vi "Drive_PositionControl.vi"(8 "error in":errorcluster, 9 "Speed limit":dbl, 10 "Right_Distance":dbl, 11 "Left_Distance":dbl) -> (0 "error out":errorcluster)   [LabVIEW 2009, in "Drive.lvlib"]
doc: "This VI implements position control of the robot drive using set speed function. It contains loop inside that runs until desired position is reached. So do not use this VI in the outer while loop directly. This VI also ramps up speed of the robot to make position control more accurate.\n\nThe VI requires desired distances to travel for both left and right sides of the robot as inputs.\nSpeed input value limits the speed of the robot during movement.\n\nTo abort the execution, use \"Drive_StopDrive\" VI and set input \"Abort?\" to true.\nTo straight forward movement, input the same value to both distances.\nTo turn on spot, input opposite values to distances.\nDifferent values will cause the robot to move along arc with some radius."
uses:
  Drive.lvlib
  <vilib>/Platform/TimedLoop/XDataNode/XDataNode.xnode
  <vilib>/Platform/TimedLoop/XDataNode/loadlvalarms.vi
  <vilib>/Platform/TimedLoop/XDataNode/timing_clust.ctl
  <vilib>/Platform/TimedLoop/XDataNode/nitl_modes.ctl
  <vilib>/Platform/TimedLoop/XDataNode/wakeup.ctl
  Drive_Utils_CalculateSpeed.vi
  Drive_ControlMode.ctl
  <vilib>/Platform/TimedLoop/XDataNode/XDNodeRunTimeDep.lvlib
  Drive_Utils.lvlib
  Utility.lvlib
panel:
  out "state out":T1
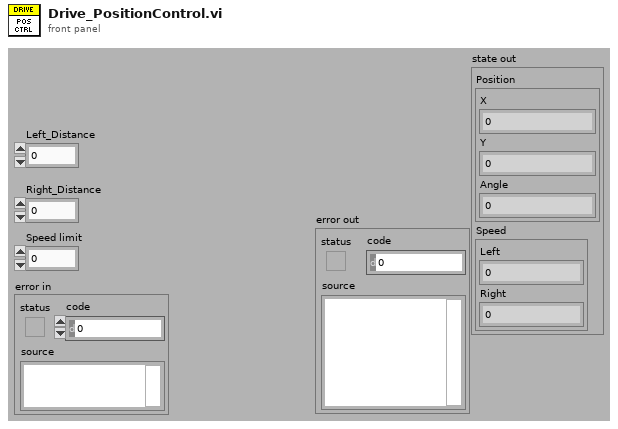
[diagram p1: front panel]
types:
  T1 = cluster{"Position":cluster{"X":dbl, "Y":dbl, "Angle":dbl}, "Speed":cluster{"Left":dbl, "Right":dbl}}
  T2 = typedef "XDNodeRunTimeDep.lvlib/timing_clust.ctl" = cluster{"Expected End [f-1]":u64, "Actual End [f-1]":u64, "Finished Late? [f-1]":bool, "Expected End [i-1]":u64, "Actual End [i-1]":u64, "Finished Late? [i-1]":bool, "Expected Start [i]":u64, "Actual Start [i]":u64, "Expected Start [f]":u64, "Actual Start [f]":u64, "Source Name":string, "Structure Name":string, "Period":i64, "Deadline":i64, "Offset":i64, "Start":i64, "Priority":i32, "Timeout":i32, "Mode":T3, "Wakeup Reason":T4, "Error":errorcluster, "Source Type":string, "Secondary Source Type":string, "Global End Time":u64, "Global Start Time":u64, "Frame Duration":u64, "Iteration Duration":u64, "Assigned CPU":i32, "I/O Scan Engine Mode":u32}
  T3 = typedef "XDNodeRunTimeDep.lvlib/nitl_modes.ctl" = enum32{"No Change", "Process missed periods, maintain original phase", "Discard missed periods, maintain original phase", "Process missed periods, ignore original phase", "Discard missed periods, ignore original phase"}
  T4 = typedef "XDNodeRunTimeDep.lvlib/wakeup.ctl" = enum32{"Normal", "Aborted", "Asynchronous wakeup", "Timing source error", "Timed loop error", "Timeout"}
  T5 = typedef "Drive.lvlib/Drive_ControlMode.ctl" = enum16{"CAN", "PWM"}
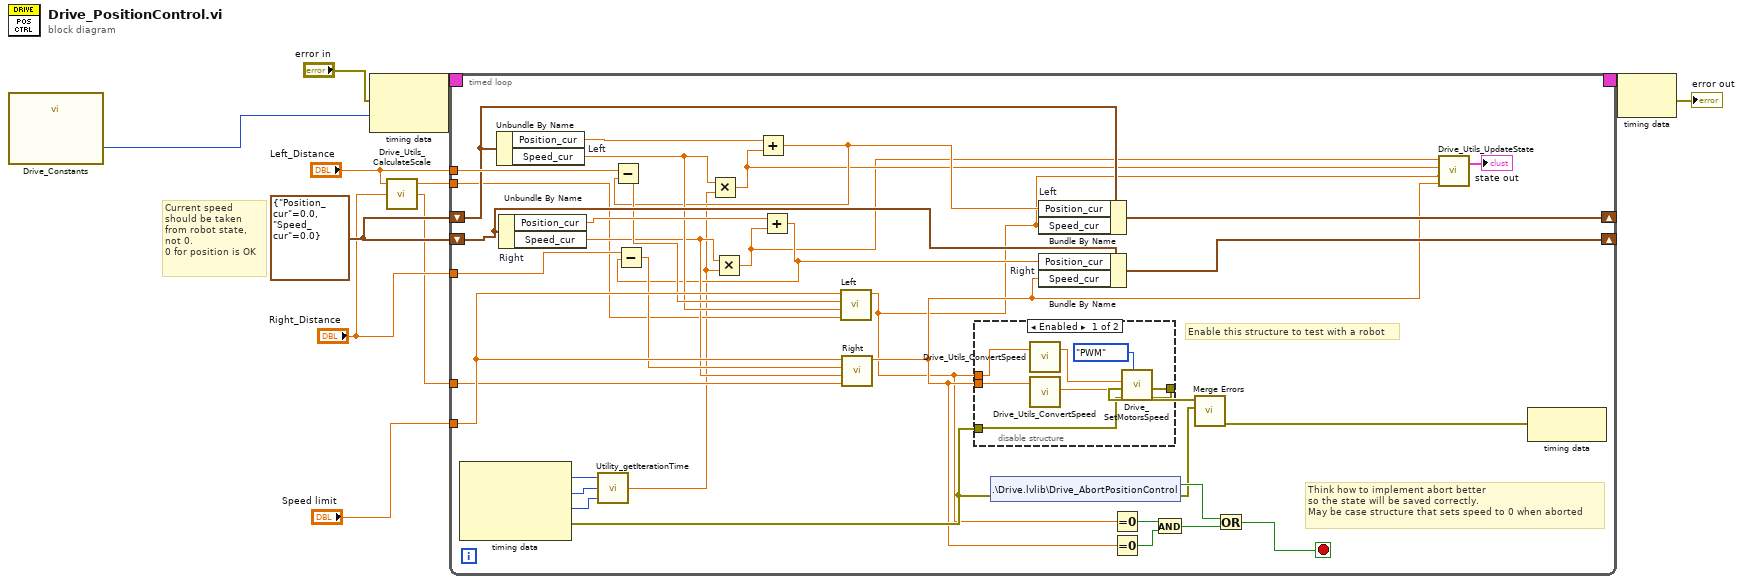
[diagram p0: block diagram]
diagram:
  w6 = cluster{"Position_cur":dbl, "Speed_cur":dbl} {"Position_cur"=0.0, "Speed_cur"=0.0}
  # "Current speed\nshould be taken\nfrom robot state,\nnot 0.\n0 for position is OK"
  n1 = call "Drive_Constants.vi"() -> ("Position control loop period (ms)"=w1:i64)  [unwired: 23 in, 4 out]
  n2 = node-c288("error in", w1) -> (w11:T2)
  n3 = call "Drive_Utils_CalculateScale.vi"("Right distance"="Right_Distance", "Left distance"="Left_Distance") -> ("Right scale"=w2:dbl, "Left scale"=w3:dbl)  [unwired: 1 in, 1 out]
  n4 = timed-loop {
    timing: w11 -> [_]
    timing-out: [_] -> w10
    tunnel: "Left_Distance" -> [w46]
    shift-right: [w43] -> _
    shift-left: w6 -> [w44]
    shift-right: [w40] -> _
    shift-left: w6 -> [w39]
    tunnel: "Right_Distance" -> [w42]
    tunnel: "Speed limit" -> [w38]
    tunnel: w3 -> [w29]
    tunnel: w2 -> [w28]
    stop <- w25 stop-if-true
    # "Enable this structure to test with a robot"
    # "Think how to implement abort better\nso the state will be saved correctly.\nMay be case structure that sets speed to 0 when aborted"
    n5 = node-c288() -> (w23:i64, w22:i64, w21:i64, w20:errorcluster)  [unwired: 1 in]
    n6 = Unbundle By Name "Left"(w44) -> ("Position_cur"=w45:dbl, "Speed_cur"=w35:dbl)
    n7 = Unbundle By Name "Right"(w39) -> ("Position_cur"=w41:dbl, "Speed_cur"=w34:dbl)
    n8 = call "Utility_getIterationTime.vi"("Duration (previous)"=w21, "End Time (previous)"=w22, "Start Time (current)"=w23) -> ("Time (Sec)"=w24:dbl)  [unwired: 1 in]
    n9 = Multiply(x=w35, y=w24) -> (x*y=w14:dbl)
    n10 = Multiply(x=w34, y=w24) -> (x*y=w13:dbl)
    n11 = Add(x=w45, y=w14) -> (x+y=w31:dbl)
    n12 = Subtract(x=w46, y=w31) -> (x-y=w37:dbl)
    n13 = Add(x=w41, y=w13) -> (x+y=w30:dbl)
    n14 = Subtract(x=w42, y=w30) -> (x-y=w36:dbl)
    n15 = call "Left"("Scaling factor"=w29, "Speed current"=w35, "delta Distance"=w37, "Speed limit"=w38) -> ("Speed"=w15:dbl)  [unwired: 6 in, 1 out]
    n16 = call "Right"("Scaling factor"=w28, "Speed current"=w34, "delta Distance"=w36, "Speed limit"=w38) -> ("Speed"=w16:dbl)  [unwired: 6 in, 1 out]
    n17 = disable-structure shown="Enabled" {
      disable-tunnel: w20 -> [w53 w54]
      disable-tunnel: [w52 w54] -> w18
      disable-tunnel: w15 -> [w51 _]
      disable-tunnel: w16 -> [w50 _]
      frame #0 {
        n18 = call "Drive_Utils_ConvertSpeed.vi"("Speed (m/s)"=w51) -> ("Speed (-1..1)"=w49:dbl)  [unwired: 1 in, 1 out]
        n19 = call "Drive_Utils_ConvertSpeed.vi"("Speed (m/s)"=w50) -> ("Speed (-1..1)"=w48:dbl)  [unwired: 1 in, 1 out]
        n20 = call "Drive_SetMotorsSpeed.vi"("ControlMode"=Drive_ControlMode."PWM", "error in"=w53, "Right_Speed"=w48, "Left_Speed"=w49) -> ("error out"=w52:errorcluster)  [unwired: 6 in, 1 out]
      }
      frame #1 {
      }
    }
    n21 = shared-variable ".\\Drive.lvlib\\Drive_AbortPositionControl"(error in=w20) -> (w27:bool, error out=w19:errorcluster)
    n22 = Bundle By Name "Left"(cluster=w44, "Position_cur"=w31, "Speed_cur"=w15) -> (w43:cluster{"Position_cur":dbl, "Speed_cur":dbl})
    n23 = Bundle By Name "Right"(cluster=w39, "Position_cur"=w30, "Speed_cur"=w16) -> (w40:cluster{"Position_cur":dbl, "Speed_cur":dbl})
    n24 = Equal To 0?(x=w15) -> (x = 0?=w33:bool)
    n25 = Equal To 0?(x=w16) -> (x = 0?=w32:bool)
    n26 = And(x=w33, y=w32) -> (x .and. y?=w26:bool)
    n27 = call <vilib>:"Merge Errors.vi"("error in 2 (no error)"=w19, "error in 1 (no error)"=w18) -> ("error out"=w17:errorcluster)  [unwired: 5 in]
    n28 = Or(x=w27, y=w26) -> (x .or. y?=w25:bool)
    n29 = call "Drive_Utils_UpdateState.vi"("delta right"=w13, "delta left"=w14, "speed left"=w15, "speed right"=w16) -> ("state out"=→"state out":T1)  [unwired: 1 in, 1 out]
    n30 = node-c288(w17) -> ()  [unwired: 1 out]
  }
  n31 = node-c288(w10) -> (→"error out":errorcluster)
